vi "Reserve Sessions with Observer.vi"(6 "timeout (ms)":i32, 7 "reservation observer":refnum<class "IReservationObserver.lvclass">, 8 "error in":errorcluster, 9 "instrument type id":string, 10 "pin or relay names":string[](array[string]), 11 "pin map context":T1) -> (0 "error out":errorcluster, 3 "session reservation out":refnum<class "Session Reservation.lvclass">)   [LabVIEW 2020, in "MeasurementLink Session Management.lvlib" / "Session Reservation.lvclass"]
doc: "Reserves session(s) based on the provided instrument type and pin information."
uses:
  Session Reservation.lvclass
  MeasurementLink Session Management Client/RPC Messages/ni_measurementlink_PinMapContext.ctl
  IReservationObserver/IReservationObserver.lvclass
  MeasurementLink Session Management Client/RPC Messages/ni_measurementlink_sessionmanagement_v1_ReserveSessionsRequest.ctl
  MeasurementLink Session Management Client/MeasurementLink Session Management Client.lvlib
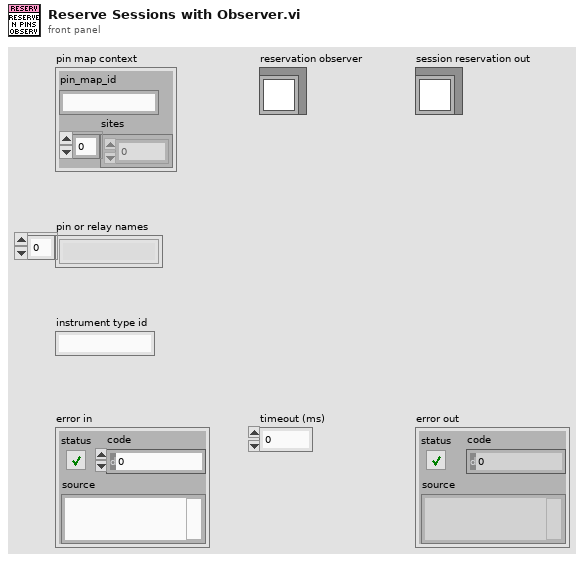
[diagram p1: front panel]
types:
  T1 = typedef "MeasurementLink Session Management Client.lvlib/ni_measurementlink_PinMapContext.ctl" = cluster{"pin_map_id":string, "sites":i32[]}
  T2 = typedef "MeasurementLink Session Management Client.lvlib/ni_measurementlink_sessionmanagement_v1_ReserveSessionsRequest.ctl" = cluster{"pin_map_context":T1, "pin_or_relay_names":string[], "instrument_type_id":string, "timeout_in_milliseconds":i32}
  T3 = typedef "MeasurementLink Session Management Client.lvlib/ni_measurementlink_sessionmanagement_v1_ReserveSessionsResponse.ctl" = cluster{"sessions":T4[]}
  T4 = typedef "MeasurementLink Session Management Client.lvlib/ni_measurementlink_sessionmanagement_v1_SessionInformation.ctl" = cluster{"session":T5, "resource_name":string, "channel_list":string, "instrument_type_id":string, "session_exists":bool, "channel_mappings":T6[]}
  T5 = typedef "MeasurementLink Session Management Client.lvlib/nidevice_grpc_Session.ctl" = cluster{"name":string}
  T6 = typedef "MeasurementLink Session Management Client.lvlib/ni_measurementlink_sessionmanagement_v1_ChannelMapping.ctl" = cluster{"pin_or_relay_name":string, "site":i32, "channel":string}
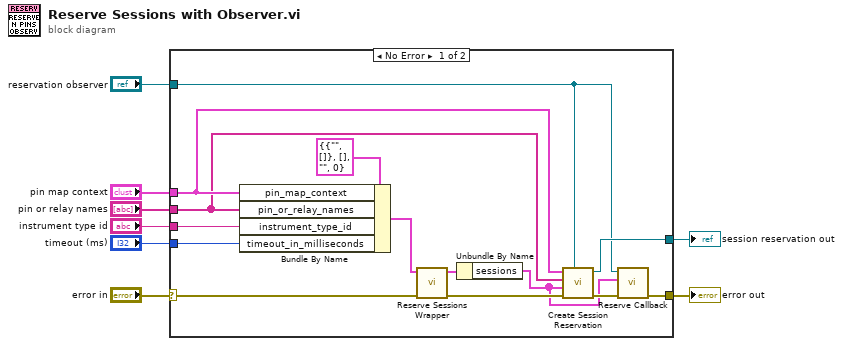
[diagram p0: block diagram]
diagram:
  n1 = case shown="No Error" "error in" {
    selector: "error in" -> [w11 w23]
    tunnel: "instrument type id" -> [w21 _]
    tunnel: "pin or relay names" -> [w16 _]
    tunnel: "timeout (ms)" -> [w20 _]
    tunnel: "pin map context" -> [w17 _]
    tunnel: [w14 w23] -> w4
    tunnel: [w18 _] -> w2
    tunnel: "reservation observer" -> [w13 _]
    frame No Error {
      n2 = Bundle By Name(cluster=T2 {"pin_map_context"={"pin_map_id"="", "sites"=[]}, "pin_or_relay_names"=[], "instrument_type_id"="", "timeout_in_milliseconds"=0} ("Request Data"), "pin_map_context"=w17, "pin_or_relay_names"=w16, "instrument_type_id"=w21, "timeout_in_milliseconds"=w20) -> (w9:T2)
      n3 = call "Reserve Sessions Wrapper.vi"("error in"=w11, "request data"=w9) -> ("error out"=w19:errorcluster, "response data"=w10:T3)  [unwired: 8 in]
      n4 = Unbundle By Name(w10) -> ("sessions"=w12:T4[])
      n5 = call "Create Session Reservation.vi"("reservation observer"=w13, "error in (no error)"=w19, "sessions"=w12, "pin or relay names"=w16, "pin map context"=w17) -> ("error out"=w15:errorcluster, "session reservation out"=w18:refnum<class "Session Reservation.lvclass">)  [unwired: 5 in]
      n6 = call-dynamic "Reserve Callback.vi"("error in"=w15, "session infos"=w12, "reservation observer in"=w13) -> ("error out"=w14:errorcluster)  [unwired: 7 in, 1 out]
    }
    frame Error {
    }
  }
  "session reservation out" <- w2
  "error out" <- w4
